vi "CheckArmAngle.vi"(10 "Tolerance  Angle Difference":dbl, 11 "Target Angle":dbl) -> (3 "Outside Tolerance":bool)   [LabVIEW 2013]
panel:
  out "Angle Difference":dbl
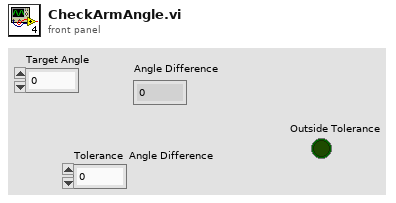
[diagram p1: front panel]
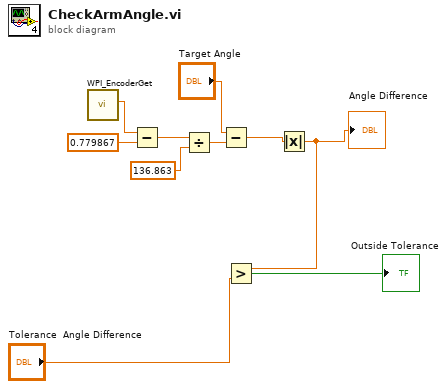
[diagram p0: block diagram]
diagram:
  n1 = call <vilib>:"WPI_EncoderGet.vi"() -> ("Distance"=w7:dbl)  [unwired: 6 in, 5 out]
  n2 = Subtract(x=w7, y=0.779867) -> (x-y=w10:dbl)
  n3 = Divide(x=w10, y=136.863) -> (x/y=w5:dbl)
  n4 = Subtract(x="Target Angle", y=w5) -> (x-y=w4:dbl)
  n5 = Absolute Value(x=w4) -> (abs(x)=w3:dbl)
  "Angle Difference" <- w3
  n6 = Greater?(x=w3, y="Tolerance  Angle Difference") -> (0:→"Outside Tolerance":bool)
